vi "Configuration Dialog Box.vi"(8 "error in (no error)":errorcluster, 11 "Configuration Setting In":T2={"offset"=0.0, "Signal Type"=enum."Sine Wave", "Amplitude"=1.0, "Frequency"=10.0, "Phase"=0.0, "Noise Amplitude "=1.0} {"Noise Amplitude" format="%.2p"; "Phase" format="%.2p"; "Frequency" format="%0.2p"; "Amplitude" format="%0.2p"; "offset" format="%0.2p"}) -> (0 "error out":errorcluster, 3 "Configuration Setting Out":T2={"offset"=0.0, "Signal Type"=enum."Sine Wave", "Amplitude"=1.0, "Frequency"=10.0, "Phase"=0.0, "Noise Amplitude "=1.0} {"Noise Amplitude" format="%.2p"; "Phase" format="%.2p"; "Frequency" format="%0.2p"; "Amplitude" format="%0.2p"; "offset" format="%0.2p"})   [LabVIEW 2020]
panel:
  in  "Noise Amplitude":dbl=1.0 format="%.2p"
  in  "Phase":dbl format="%.2p"
  in  "Frequency":dbl=10.0 format="%0.2p"
  in  "Amplitude":dbl=1.0 format="%0.2p"
  in  "Signal Type":T1(ring)
  in  "offset":dbl format="%0.2p"
  in  "Cancel":bool
  in  "Ok":bool
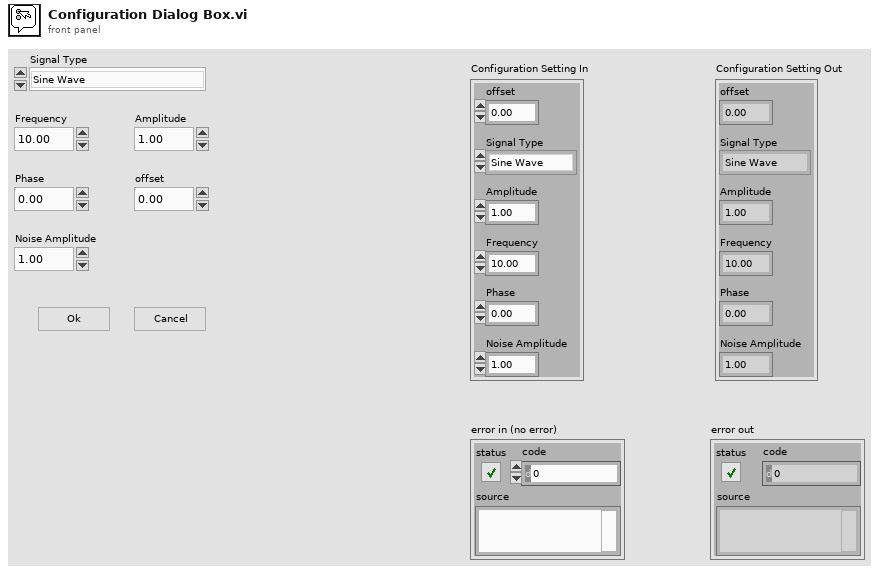
[diagram p1: front panel]
types:
  T1 = enum16{"Sine Wave", "Triangle Wave", "Square Wave", "Sawtooth Wave"}
  T2 = cluster{"offset":dbl, "Signal Type":enum16{"Sine Wave", "Triangle Wave", "Square Wave", "Sawtooth Wave"}, "Amplitude":dbl, "Frequency":dbl, "Phase":dbl, "Noise Amplitude ":dbl}
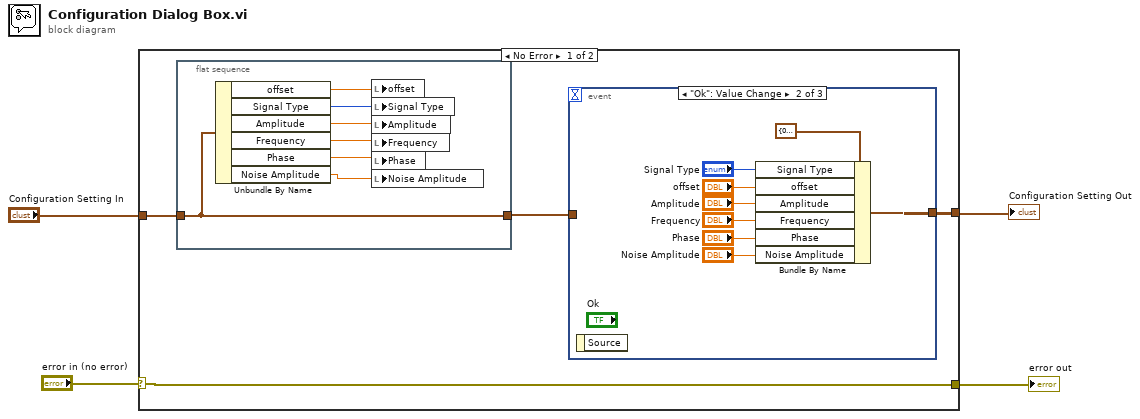
[diagram p0: block diagram]
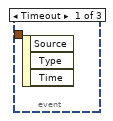
[diagram p2: hidden frame]
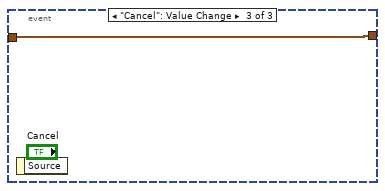
[diagram p3: hidden frame]
diagram:
  n1 = case shown="No Error" "error in (no error)" {
    selector: "error in (no error)" -> [w8 _]
    tunnel: [w8 _] -> w3
    tunnel: "Configuration Setting In" -> [w6 _]
    tunnel: [w7 _] -> w1
    frame No Error {
      n2 = flat-sequence {
        tunnel: w6 -> [w9]
        tunnel: [w9] -> w5
        frame #0 {
          n3 = Unbundle By Name(w9) -> ("offset"=w15:dbl, "Signal Type"=w14:T1, "Amplitude"=w13:dbl, "Frequency"=w12:dbl, "Phase"=w11:dbl, "Noise Amplitude"=w10:dbl)
          n4 = local write "offset"(w15) -> ()
          n5 = local write "Signal Type"(w14) -> ()
          n6 = local write "Amplitude"(w13) -> ()
          n7 = local write "Frequency"(w12) -> ()
          n8 = local write "Phase"(w11) -> ()
          n9 = local write "Noise Amplitude"(w10) -> ()
        }
      }
      n10 = event shown="[1] \"Ok\": Value Change" {
        selector: _ -> [_ _ _]
        dyn-events: _ -> [_ _ _]
        timeout: _ -> [_ _ _]
        tunnel: [_ w16 w24] -> w7
        tunnel: w5 -> [_ _ w24]
        event Timeout {
          n11 = event-data() -> ()  [unwired: 1 in, 3 out]
        }
        event "Ok": Value Change {
          n12 = event-data() -> ()  [unwired: 1 in, 1 out]
          n13 = Bundle By Name(cluster=T2 {"offset"=0.0, "Signal Type"=enum."Sine Wave", "Amplitude"=1.0, "Frequency"=10.0, "Phase"=0.0, "Noise Amplitude "=1.0} ("Configuration Setting Out"), "Signal Type"="Signal Type", "offset"="offset", "Amplitude"="Amplitude", "Frequency"="Frequency", "Phase"="Phase", "Noise Amplitude"="Noise Amplitude") -> (w16:T2)
        }
        event "Cancel": Value Change {
          n14 = event-data() -> ()  [unwired: 1 in, 1 out]
        }
      }
    }
    frame Error {
    }
  }
  "Configuration Setting Out" <- w1
  "error out" <- w3
